vi "2L13-ech2D_tab1D_pop_moy_et_ec.vi"(2 "Nb Ech Taille n":sgl[][](array[numeric])) -> (1 "m":dbl caption="moyenne" format="%0.2f", 4 "x_bar (1D)":dbl[](array[numeric]), 5 "S pop":dbl caption="S pop estimé" format="%0.2f", 6 "s ech":dbl caption="s" format="%0.2f", 7 "ech 1D":dbl[](array[numeric]), 8 "r (1D)":dbl[](array[numeric]), 9 "S Dem éch de taille n":dbl format="%.2f", 10 "s (1D)":dbl[](array[numeric]))   [LabVIEW 2010, in "lv_02.lvlib"]
doc: "Ce VI permet de traiter une série d'achantillons contenus dans un tableau 2D de Nb échantillons (lignes) de taille n (colonnes). En sortie on retrouve un tableau 1D contenant les Nb*n valeurs mesurées, 3 tableaux 1D des moyennes, étendues et écart-type d'échantillon. La taille des 3 tableaux 1D est Nb.\nS pop estimé est l'écart-type calculé de la population à partire des données 2D vues comme un échantillon.\ns est l'écart-type calculé des données 2D sans pondération.\nDonc si vos données 2D sont une population et non un échantillon, l'écart-type de cette population est s"
uses:
  lv_02.lvlib
  <vilib>/Analysis/NI_AALBase.lvlib
panel:
  out "élément":i32
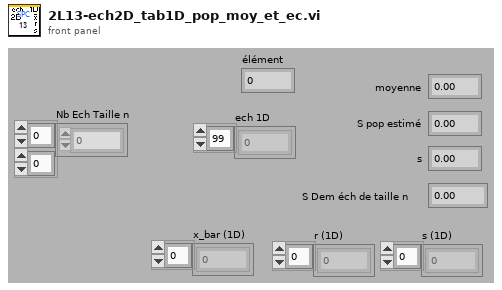
[diagram p1: front panel]
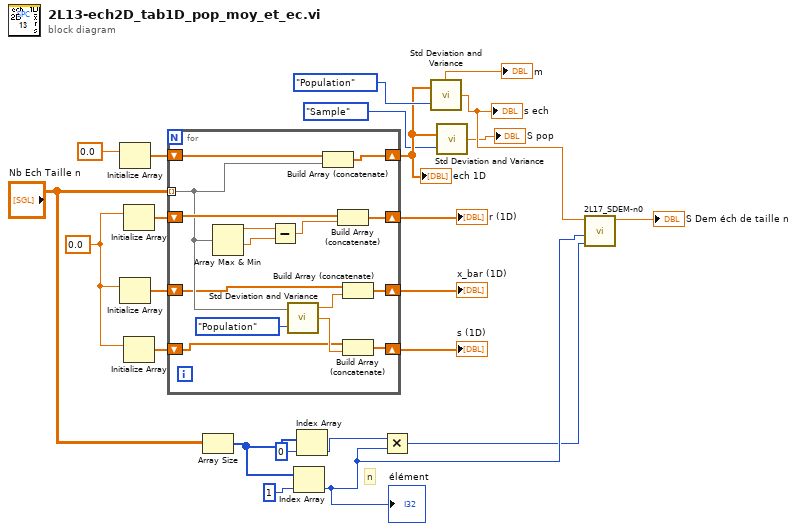
[diagram p0: block diagram]
diagram:
  w23 = 0.0 ("Nouvel élément")
  # "n"
  n1 = Initialize Array(0.0 ("Nouvel élément")) -> (w19:dbl[])  [unwired: 1 in]
  n2 = Initialize Array(w23) -> (w15:dbl[])  [unwired: 1 in]
  n3 = Initialize Array(w23) -> (w16:dbl[])  [unwired: 1 in]
  n4 = Initialize Array(w23) -> (w21:dbl[])  [unwired: 1 in]
  n5 = for {
    tunnel: "Nb Ech Taille n" -> [w30] mode=indexing
    shift-right: [w37] -> w8
    shift-left: w19 -> [w38]
    shift-right: [w33] -> w18
    shift-left: w15 -> [w26]
    shift-right: [w32] -> w17
    shift-left: w16 -> [w34]
    shift-right: [w24] -> w22
    shift-left: w21 -> [w25]
    n6 = Array Max & Min(array=w30) -> (max value=w36:sgl, min value=w35:sgl)  [unwired: 2 out]
    n7 = Subtract(x=w36, y=w35) -> (x-y=w31:sgl)
    n8 = call <vilib>:"Std Deviation and Variance.vi"("X"=w30, "Weighting (Sample)"=enum16{"Sample", "Population"}."Population") -> ("mean"=w29:dbl, "standard deviation"=w28:dbl)  [unwired: 1 out]
    n9 = Build Array (concatenate)(w38, w30) -> (w37:dbl[])
    n10 = Build Array (concatenate)(w34, w31) -> (w32:dbl[])
    n11 = Build Array (concatenate)(w26, w29) -> (w33:dbl[])
    n12 = Build Array (concatenate)(w25, w28) -> (w24:dbl[])
  }
  "s (1D)" <- w22
  "x_bar (1D)" <- w18
  "r (1D)" <- w17
  "ech 1D" <- w8
  n13 = Array Size(array="Nb Ech Taille n") -> (size(s)=w5:i32[])
  n14 = Index Array(array=w5, index=1 ("indice")) -> (element=w2:i32)
  "élément" <- w2
  n15 = Index Array(array=w5, index=0 ("indice")) -> (element=w3:i32)
  n16 = Multiply(x=w3, y=w2) -> (x*y=w1:i32)
  n17 = call <vilib>:"Std Deviation and Variance.vi"("X"=w8, "Weighting (Sample)"=enum16{"Sample", "Population"}."Population") -> ("mean"=→"m":dbl, "standard deviation"=w12:dbl)  [unwired: 1 out]
  "s ech" <- w12
  n18 = call <vilib>:"Std Deviation and Variance.vi"("X"=w8, "Weighting (Sample)"=enum16{"Sample", "Population"}."Sample") -> ("standard deviation"=→"S pop":dbl)  [unwired: 2 out]
  n19 = call "2L17_SDEM-n0.vi"("N"=w1, "n"=w2, "s"=w12) -> ("S DEM"=→"S Dem éch de taille n":dbl)  [unwired: 6 in, 2 out]
